vi "Read_user_key.vi"(8 "Error in":errorcluster, 10 "Senha":string, 11 "User":string) -> (0 "Error out":errorcluster, 1 "x = y?":bool, 2 "Key":string, 3 "Dados Válidos":bool)   [LabVIEW 2016]
uses:
  <vilib>/Utility/config.llb/Read Key (String).vi
  <vilib>/Utility/config.llb/NI_LVConfig.lvlib
panel:
  in  "configuration file path":path=path "C:/Users/Lucas Oliveira/Desktop/Software_TCC/Config/Config.ini"
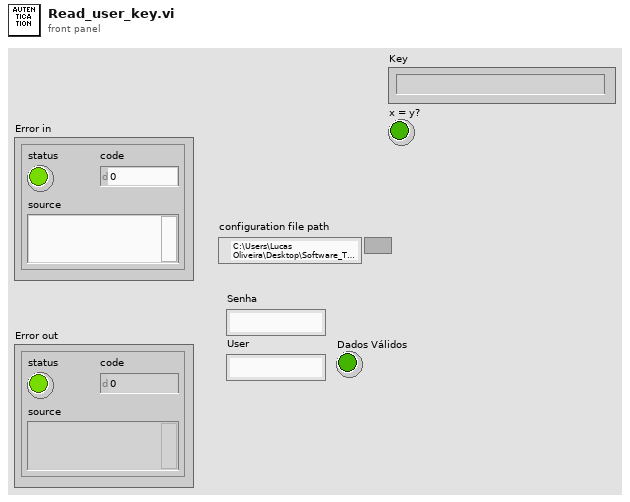
[diagram p1: front panel]
types:
  T1 = typedef "NI_LVConfig.lvlib/Config Data RefNum.ctl" = refnum<k1>
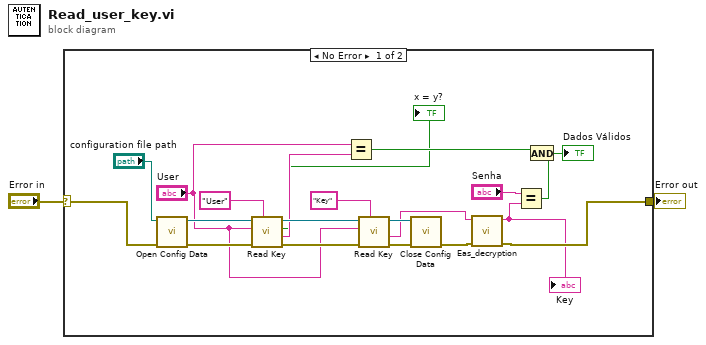
[diagram p0: block diagram]
diagram:
  n1 = case shown="No Error" "Error in" {
    selector: "Error in" -> [w14 w24]
    tunnel: [w12 w24] -> w1
    frame No Error {
      n2 = call <vilib>:"Open Config Data.vi"("error in (no error)"=w14, "configuration file path"="configuration file path") -> ("error out"=w23:errorcluster, "refnum"=w22:T1)  [unwired: 7 in, 1 out]
      n3 = call-poly <vilib>:"Read Key.vi"("section"="User", "error in (no error)"=w23, "key"="User", "refnum"=w22) -> ("error out"=w19:errorcluster, "value"=w8:string, "found?"=→"x = y?":bool, "refnum out"=w18:T1)  [unwired: 4 in]
      n4 = Equal?(x="User", y=w8) -> (x = y?=w5:bool)
      n5 = call-poly <vilib>:"Read Key.vi"("section"="Key", "error in (no error)"=w19, "key"="User", "refnum"=w18) -> ("error out"=w17:errorcluster, "value"=w11:string, "refnum out"=w16:T1)  [unwired: 4 in, 1 out]
      n6 = call <vilib>:"Close Config Data.vi"("error in (no error)"=w17, "refnum"=w16) -> ("error out"=w13:errorcluster)  [unwired: 8 in, 1 out]
      n7 = call "Eas_decryption.vi"("Error In"=w13, "Key"=w11) -> ("error out"=w12:errorcluster, "Key"=w10:string)  [unwired: 8 in]
      "Key" <- w10
      n8 = Equal?(x="Senha", y=w10) -> (x = y?=w6:bool)
      n9 = And(x=w5, y=w6) -> (x .and. y?=→"Dados Válidos":bool)
    }
    frame Error {
    }
  }
  "Error out" <- w1
